vi "updateFromOdometry.vi"(8 "CC":T1, 9 "P":dbl[][](array[numeric]), 10 "dX":dbl[](array[numeric]), 11 "X":dbl[](array[numeric])) -> (2 "P out":dbl[][](array[numeric]), 3 "X out":dbl[](array[numeric]))   [LabVIEW 2009, in "LV_SLAM.lvlib"]
uses:
  LV_SLAM.lvlib
  <vilib>/Analysis/Matrix/Datatypes/RealMatrix.ctl
  <vilib>/Analysis/Matrix/Numeric/Add/Add - RM,RM.vi
  <vilib>/Analysis/Matrix/Numeric/Multiply/Multiply - RM,RM.vi
  <vilib>/Analysis/Matrix/Numeric/Conversions/Array To Matrix - RA2.vi
  <vilib>/Analysis/Matrix/NI_Matrix.lvlib
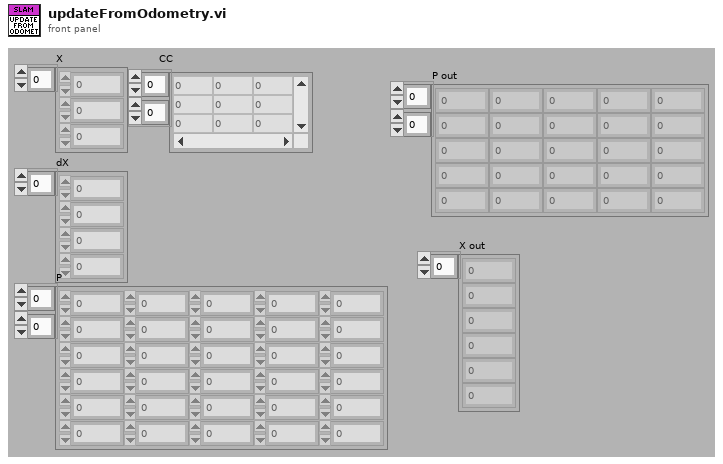
[diagram p1: front panel]
types:
  T1 = typedef "NI_Matrix.lvlib/RealMatrix.ctl" = dbl[][]
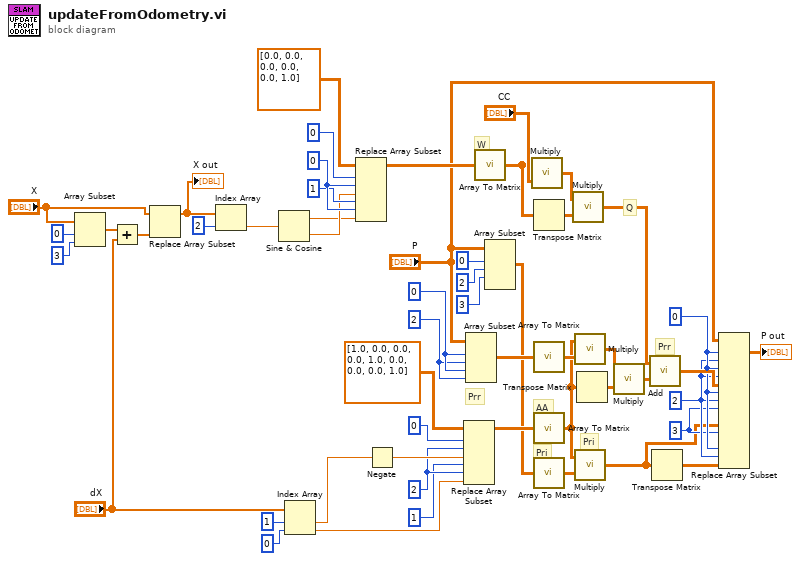
[diagram p0: block diagram]
diagram:
  w4 = 3
  w5 = 2 ("row N")
  w6 = 0 ("row 1")
  w21 = 2 ("row N")
  w22 = 0 ("row 1")
  w32 = 0 ("disabled index (col)")
  w39 = 2 ("disabled index (col)")
  # "Pri"
  # "Prr"
  # "Pri"
  # "Prr"
  # "Q"
  # "W"
  # "AA"
  n1 = Array Subset(array="X", index=0, length=3) -> (w49:dbl[])
  n2 = Add(x=w49, y="dX") -> (x+y=w48:dbl[])
  n3 = Replace Array Subset(array="X", new element=w48) -> (w36:dbl[])  [unwired: 1 in]
  "X out" <- w36
  n4 = Index Array(array=w36, index=2) -> (element=w34:dbl)
  n5 = Sine & Cosine(0:w34) -> (1:w28:dbl, 2:w29:dbl)
  n6 = Index Array(array="dX", index #1=1 ("index"), index #2=0 ("index")) -> (element #1=w44:dbl, element #2=w40:dbl)
  n7 = Replace Array Subset(array=dbl[][] [[0.0, 0.0], [0.0, 0.0], [0.0, 1.0]] ("P"), new element #1=w29, index (row) #1=0 ("disabled index (row)"), index (col) #1=w32, new element #2=w28, index (row) #2=1 ("disabled index (row)"), index (col) #2=w32) -> (w27:dbl[][])
  n8 = Negate(x=w44) -> (-x=w41:dbl)
  n9 = Replace Array Subset(array=dbl[][] [[1.0, 0.0, 0.0], [0.0, 1.0, 0.0], [0.0, 0.0, 1.0]] ("P"), new element #1=w41, index (row) #1=0 ("index (row)"), index (col) #1=w39, new element #2=w40, index (row) #2=1 ("disabled index (row)"), index (col) #2=w39) -> (w37:dbl[][])
  n10 = Array Subset(array="P", index (row)=w22, length (row)=w21, index (col)=w22, length (col)=w21) -> (w17:dbl[][])
  n11 = call-poly <vilib>:"Array To Matrix.vi"("Real 2D Array"=w27) -> ("Real Matrix"=w25:T1)
  n12 = Array Subset(array="P", index (row)=0 ("row 1"), length (row)=2 ("row N"), index (col)=3 ("column 1")) -> (w10:dbl[][])  [unwired: 1 in]
  n13 = call-poly <vilib>:"Multiply.vi"("Real Matrix B"="CC", "Real Matrix A"=w25) -> ("A * B"=w23:T1)
  n14 = Transpose Matrix(1:w25) -> (0:w24:T1)
  n15 = call-poly <vilib>:"Array To Matrix.vi"("Real 2D Array"=w17) -> ("Real Matrix"=w16:T1)
  n16 = call-poly <vilib>:"Array To Matrix.vi"("Real 2D Array"=w37) -> ("Real Matrix"=w11:T1)
  n17 = call-poly <vilib>:"Array To Matrix.vi"("Real 2D Array"=w10) -> ("Real Matrix"=w9:T1)
  n18 = call-poly <vilib>:"Multiply.vi"("Real Matrix B"=w24, "Real Matrix A"=w23) -> ("A * B"=w13:T1)
  n19 = call-poly <vilib>:"Multiply.vi"("Real Matrix B"=w16, "Real Matrix A"=w11) -> ("A * B"=w15:T1)
  n20 = call-poly <vilib>:"Multiply.vi"("Real Matrix B"=w9, "Real Matrix A"=w11) -> ("A * B"=w3:T1)
  n21 = Transpose Matrix(1:w11) -> (0:w14:T1)
  n22 = call-poly <vilib>:"Multiply.vi"("Real Matrix B"=w14, "Real Matrix A"=w15) -> ("A * B"=w12:T1)
  n23 = call-poly <vilib>:"Add.vi"("Real Matrix B"=w12, "Real Matrix A"=w13) -> ("A + B"=w7:T1)
  n24 = Transpose Matrix(1:w3) -> (0:w2:T1)
  n25 = Replace Array Subset(array="P", new element #1=w7, index (dim 0) #1=w6, index (dim 1) #1=w5, index (dim 2) #1=w6, index (dim 3) #1=w5, new element #2=w3, index (dim 0) #2=w6, index (dim 1) #2=w5, index (dim 2) #2=w4, new element #3=w2, index (dim 0) #3=w4, index (dim 2) #3=w6, index (dim 3) #3=w5) -> (→"P out":T1)  [unwired: 2 in]
